vi "Write UI VI Ref.vi"(8 "error in (no error)":errorcluster, 10 "UI VI Ref":refnum<vi>, 11 "ViewableActor in":refnum<class "ViewableActor.lvclass">) -> (0 "error out":errorcluster, 3 "ViewableActor out":refnum<class "ViewableActor.lvclass">)   [LabVIEW 2014, in "ViewableActor.lvlib" / "ViewableActor.lvclass"]
uses:
  ViewableActor.lvclass
  ViewableActor.lvclass/ViewableActor.ctl
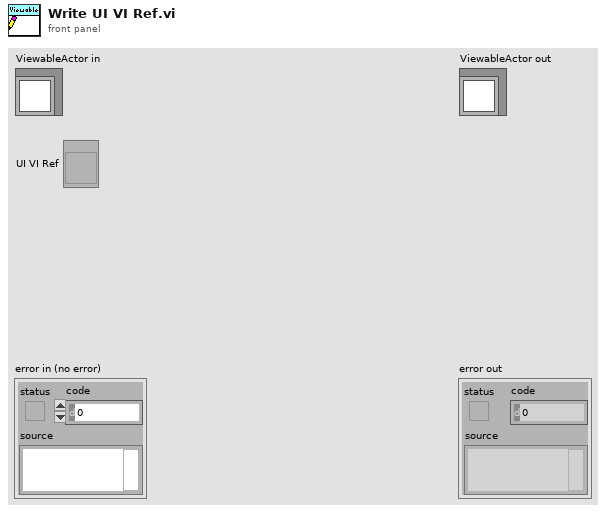
[diagram p1: front panel]
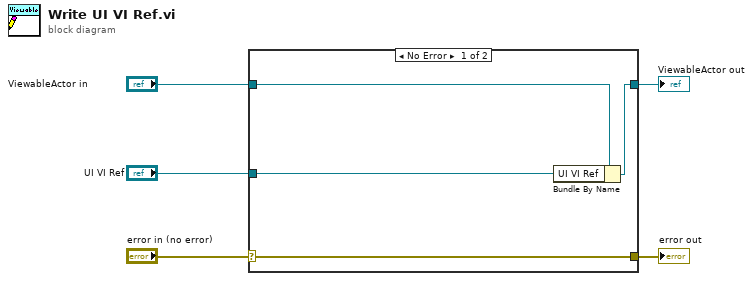
[diagram p0: block diagram]
diagram:
  n1 = case shown="No Error" "error in (no error)" {
    selector: "error in (no error)" -> [w9 w10]
    tunnel: [w9 w10] -> w4
    tunnel: [w7 w11] -> w2
    tunnel: "ViewableActor in" -> [w8 w11]
    tunnel: "UI VI Ref" -> [w6 _]
    frame No Error {
      n2 = Bundle By Name(cluster=w8, "UI VI Ref"=w6) -> (w7:refnum<class "ViewableActor.lvclass">)
    }
    frame Error {
    }
  }
  "error out" <- w4
  "ViewableActor out" <- w2
